vi "ToLabVIEW_Wrap.vi"(4 "TypeMap in":refnum<class "TypeMap.lvclass">, 8 "error in (no error)":errorcluster, 10 "DbRow":variant, 11 "TargetObject In":refnum<class>) -> (0 "error out":errorcluster, 3 "Object Out":refnum<class>)   [LabVIEW 2020, in "ORM.lvlib" / "TypeMap.lvclass"]
uses:
  TypeMap.lvclass
  <vilib>/Viviota/shared/ORM_lib.lvlibp/ObjectMap/ObjectMap.lvclass
  TypeMap.lvclass/TypeMap.ctl
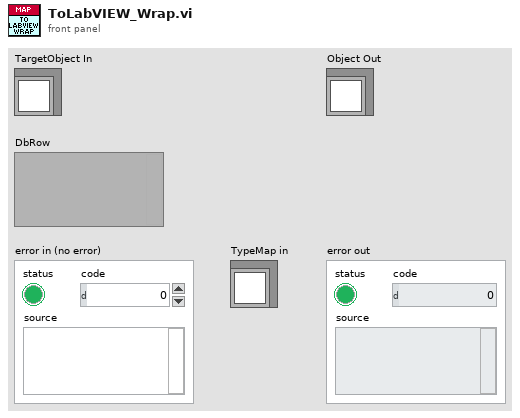
[diagram p1: front panel]
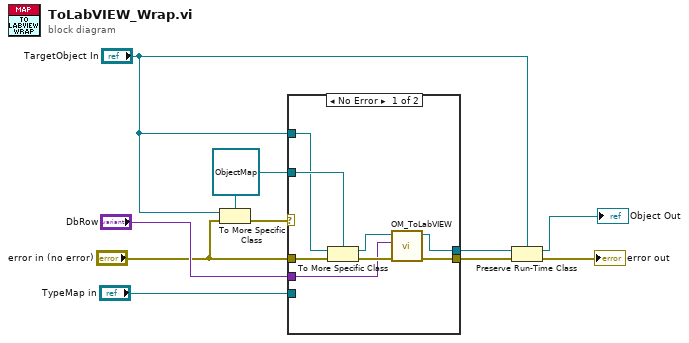
[diagram p0: block diagram]
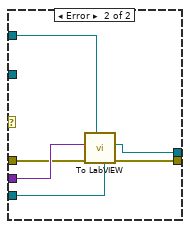
[diagram p2: hidden frame]
diagram:
  w1 = refnum<class "ObjectMap.lvclass"> refnum ("ORM_lib.lvlibp:ObjectMap")
  n1 = To More Specific Class(target class=w1, reference="TargetObject In", error in="error in (no error)") -> (error out=w2:errorcluster)  [unwired: 1 out]
  n2 = case shown="No Error" w2 {
    tunnel: "TypeMap in" -> [_ w24]
    tunnel: "DbRow" -> [w11 w23]
    tunnel: [w17 w22] -> w8
    tunnel: [w16 w21] -> w6
    tunnel: "error in (no error)" -> [w18 w20]
    tunnel: "TargetObject In" -> [w13 w19]
    tunnel: w1 -> [w14 _]
    frame No Error {
      n3 = To More Specific Class(target class=w14, reference=w13, error in=w18) -> (specific class reference=w12:refnum<class "ObjectMap.lvclass">, error out=w15:errorcluster)
      n4 = call-dynamic "OM_ToLabVIEW.vi"("error in (no error)"=w15, "DbRow"=w11, "ObjectMap in"=w12) -> ("error out"=w17:errorcluster, "ObjectMap out"=w16:refnum<class "ObjectMap.lvclass">)  [unwired: 6 in, 1 out]
    }
    frame Error {
      n5 = call-dynamic "To LabVIEW.vi"("TypeMap in"=w24, "ExpectedType"=w19, "error in (no error)"=w20, "DbRow"=w23) -> ("error out"=w22:errorcluster, "Value"=w21:refnum<class>)  [unwired: 6 in]
    }
  }
  n6 = Preserve Run-Time Class(object in=w6, error in=w8, 2:"TargetObject In") -> (object out=→"Object Out":refnum<class>, error out=→"error out":errorcluster)
